vi "VisualizeGradientProfile.vi"(9 "Image Src":T1, 10 "ExitExternalPrograms":refnum<notifier>, 11 "UpdateGradientProfile":refnum<notifier>) -> ()   [LabVIEW 2021]
uses:
  <vilib>/vision/Image Controls.llb/IMAQ Image.ctl
  <vilib>/vision/NI_Vision_Development_Module.lvlib
panel:
  out "RT Normalized Gradient Intensity Profile":sgl[](graph)
  out "error out":errorcluster
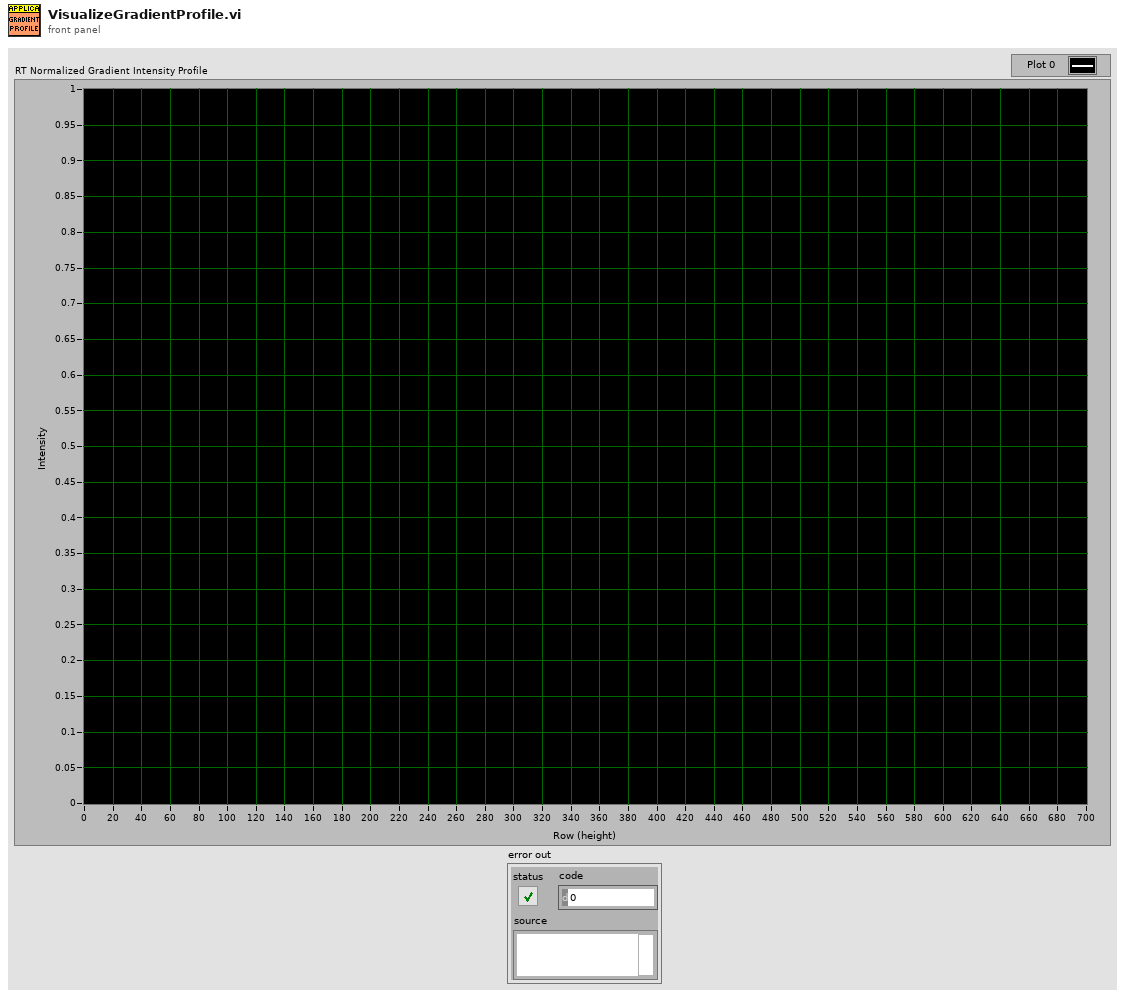
[diagram p1: front panel]
types:
  T1 = typedef "IMAQ Image.ctl" = refnum<image>
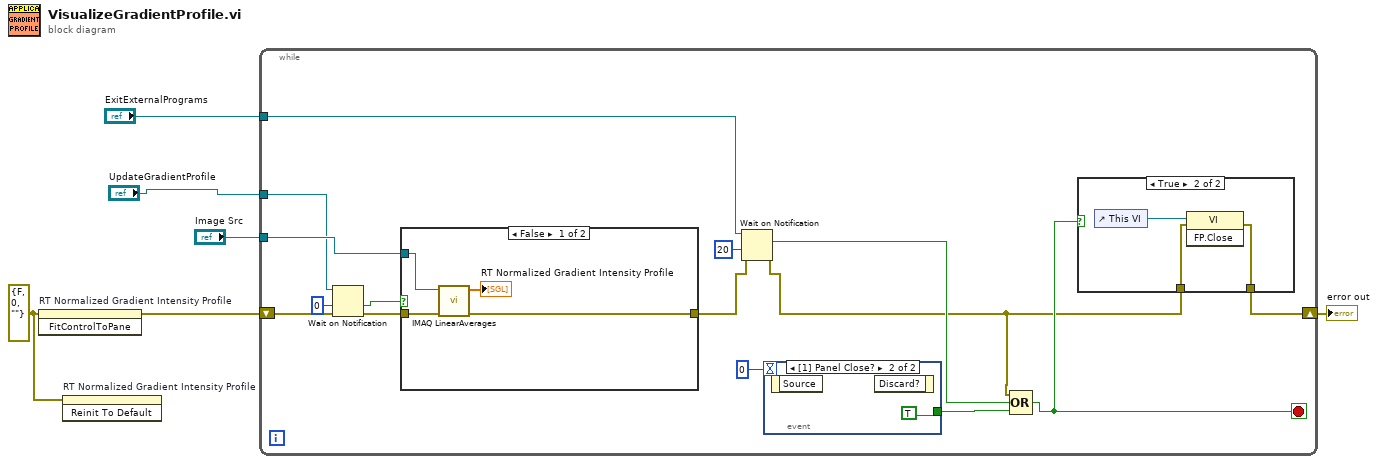
[diagram p0: block diagram]
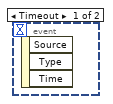
[diagram p4: hidden frame]
diagram:
  w1 = errorcluster {"status"=FALSE, "code"=0, "source"=""} ("error in (no error)")
  n1 = invoke on="RT Normalized Gradient Intensity Profile" class="WFGraph (strict)" method="FitControlToPane"(error in=w1) -> (error out=w6:errorcluster)  [unwired: 2 in, 2 out]
  n2 = invoke on="RT Normalized Gradient Intensity Profile" class="WFGraph (strict)" method="Reinit To Default"(error in=w1) -> ()  [unwired: 2 in, 3 out]
  n3 = while {
    shift-right: [w7] -> w2
    shift-left: w6 -> [w21]
    tunnel: "Image Src" -> [w19]
    tunnel: "UpdateGradientProfile" -> [w15]
    tunnel: "ExitExternalPrograms" -> [w14]
    stop <- w9 stop-if-true
    n4 = Wait on Notification(notifier=w15, timeout in ms (-1)=0, error in (no error)=w21) -> (timed out?=w16:bool, error out=w20:errorcluster)  [unwired: 1 in, 2 out]
    n5 = case shown="False" w16 {
      tunnel: w20 -> [w28 w30]
      tunnel: w19 -> [w27 _]
      tunnel: [w26 w30] -> w10
      frame False {
        n6 = call "IMAQ LinearAverages"("error in (no error)"=w28, "Image Src"=w27) -> ("error out"=w26:errorcluster, "Y Axis Averages"=→"RT Normalized Gradient Intensity Profile":sgl[])  [unwired: 5 in, 3 out]
      }
      frame True {
      }
    }
    n7 = Wait on Notification(notifier=w14, timeout in ms (-1)=20, error in (no error)=w10) -> (notification=w11:bool, error out=w8:errorcluster)  [unwired: 1 in, 2 out]
    n8 = event shown="[1] Panel Close?" {
      selector: _ -> [_ _]
      dyn-events: _ -> [_ _]
      timeout: 0 -> [_ _]
      tunnel: [_ TRUE] -> w12
      event Timeout {
        n9 = event-data() -> ()  [unwired: 1 in, 3 out]
      }
      event Panel Close? {
        n10 = event-data() -> ()  [unwired: 1 in, 1 out]
        n11 = event-data() -> ()  [unwired: 2 in, 1 out]
      }
    }
    n12 = Compound Arithmetic op=OR(w8, w11, w12) -> (w9:bool)
    n13 = case shown="True" w9 {
      tunnel: w8 -> [w22 w24]
      tunnel: [w22 w23] -> w7
      frame False {
      }
      frame True {
        n14 = control-ref of="This VI"() -> (w25:refnum<vi>)
        n15 = invoke class="VI" method="FP.Close"(reference=w25, error in=w24) -> (error out=w23:errorcluster)  [unwired: 1 in, 2 out]
      }
    }
  }
  "error out" <- w2
